vi "UIRef.vi"(8 "error in":errorcluster, 11 "Tag Bus Web Interface editor node in":refnum<class "Tag Bus Web Interface editor node.lvclass">) -> (0 "error out":errorcluster, 2 "VI refnum":refnum<vi>, 3 "Tag Bus Web Interface editor node out":refnum<class "Tag Bus Web Interface editor node.lvclass">)   [LabVIEW 2013, in "Tag Bus Web Interface editor node.lvclass"]
uses:
  Tag Bus Web Interface editor node.lvclass
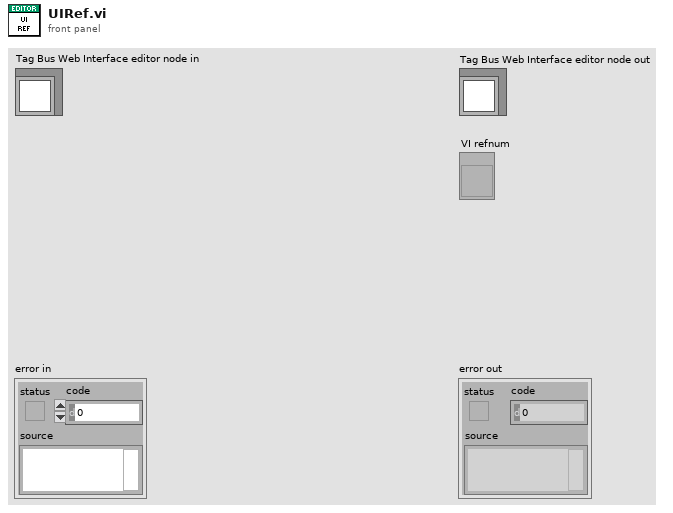
[diagram p1: front panel]
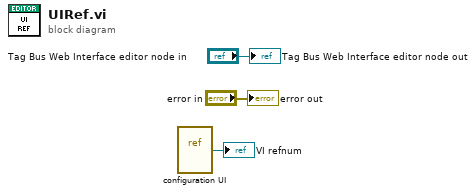
[diagram p0: block diagram]
diagram:
  n1 = vi-ref "configuration UI.vi"() -> (→"VI refnum":refnum<vi>)
  "error out" <- "error in"
  "Tag Bus Web Interface editor node out" <- "Tag Bus Web Interface editor node in"
